vi "MEASURE_hysteresis_multiple_gate_Raman_all 2450.vi"() -> ()   [LabVIEW 2020]
uses:
  <vilib>/Utility/file.llb/Write To Spreadsheet File (DBL).vi
  C/Program Files/National Instruments/LabVIEW 2016/instr.lib/Stanford Research 830/Stanford Research 830.lvlib
  C/Program Files/National Instruments/LabVIEW 2016/instr.lib/Keithley 2450/Keithley 2450.lvlib
panel:
  out "back gate leaking":string="1.162721E-12\n"
  in  "Compliance  Level (1uA)":dbl=1e-09
  in  "Function (0: Volts) 3":u16(ring) items=["Volts", "Current", "Resistance"]
  in  "topgate-off set":dbl=3.0
  in  "0ff set{T}/no off set[F]":bool
  out "XY Graph 4":cluster{dbl[], dbl[]}(graph)
  out "XY Graph 3":cluster{dbl[], dbl[]}(graph)
  out "bottom gate voltage":dbl=0.22 format="%#_13g"
  in  "backgate address":refnum<visa-resource-name>="GPIB0::18::INSTR"
  in  "bottom gate thickness":dbl=30.0
  in  "top gate thickness":dbl=10.0
  in  "pure field (T)/pure doping (F)":bool=TRUE
  out "loop run":i32=1
  in  "loop #":i32=1
  in  "Save data or not":bool
  in  "path (folder + filename)":string="C:\\Users\\User\\Data\\Jason\\03282019\\ pure_bottom_high_6v_rato3 with light2"
  in  "Clear Plot":bool
  out "LOCKIN Measurement":dbl
  in  "Parameter (1: X)":u16(ring)=3 items=["X"=1, "Y"=2, "R"=3, "Theta"=4, "Channel 1"=5, "Channel 2"=6, "Aux In 1"=7, "Aux In 2"=8, "Aux In 3"=9, "Aux In 4"=10]
  out "top gate voltage":dbl=0.22 format="%#_13g"
  out "top gate leaking":string="-2.408176E-13\n"
  in  "GATE STEP(mv)":i32=50
  in  "GATE Low Value (default 0)":dbl
  in  "GATE High Value":dbl=0.5
  in  "Function (0: Volts) 2":u16(ring) items=["Volts", "Current", "Resistance"]
  in  "Source Compaliance":dbl=1e-09
  in  "topgate address":refnum<visa-resource-name>="GPIB0::18::INSTR"
  in  "SD stabilization(S) 2":dbl=0.3 format="%#_13g"
  in  "Sine Output Amplitude (1 V) 2":dbl=0.02
  in  "GATE / SD stablization 3":dbl=0.3 format="%#_13g"
  in  "frequency":dbl=50.0 format="%#_13g"
  in  "Input Connection (0: Single-Ended Voltage)":u16(ring)=1 items=["Single-Ended Voltage", "Differential Voltage", "1 MOhm Current Gain", "100 MOhm Current Gain"]
  in  "LOCKIN address":refnum<visa-resource-name>="GPIB0::8::INSTR"
  # "Gate2450 (back) Setting"
  # "Lock-in"
  # "Gate2450(top) Setting"
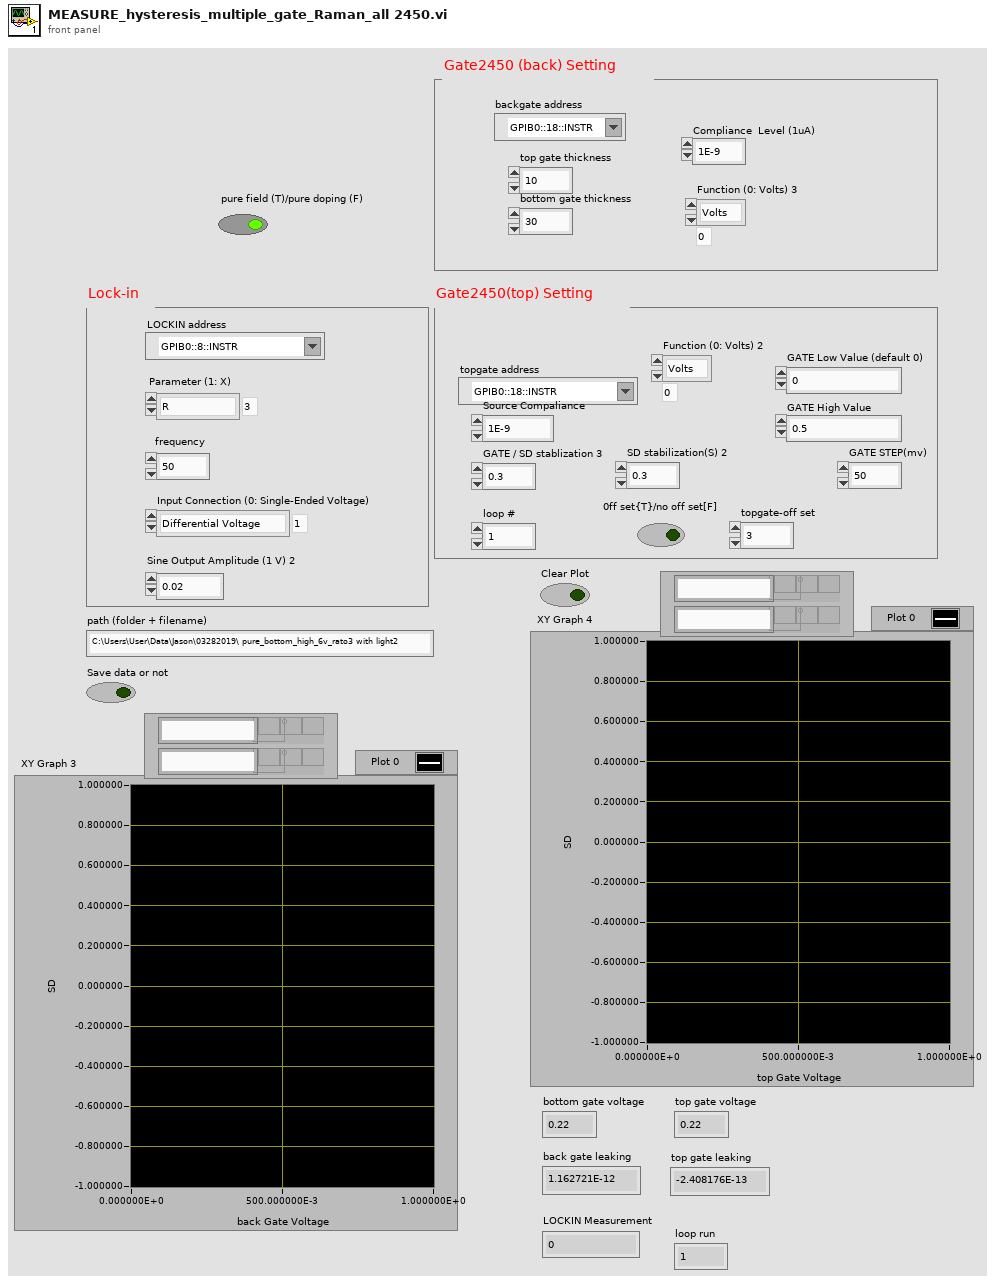
[diagram p1: front panel]
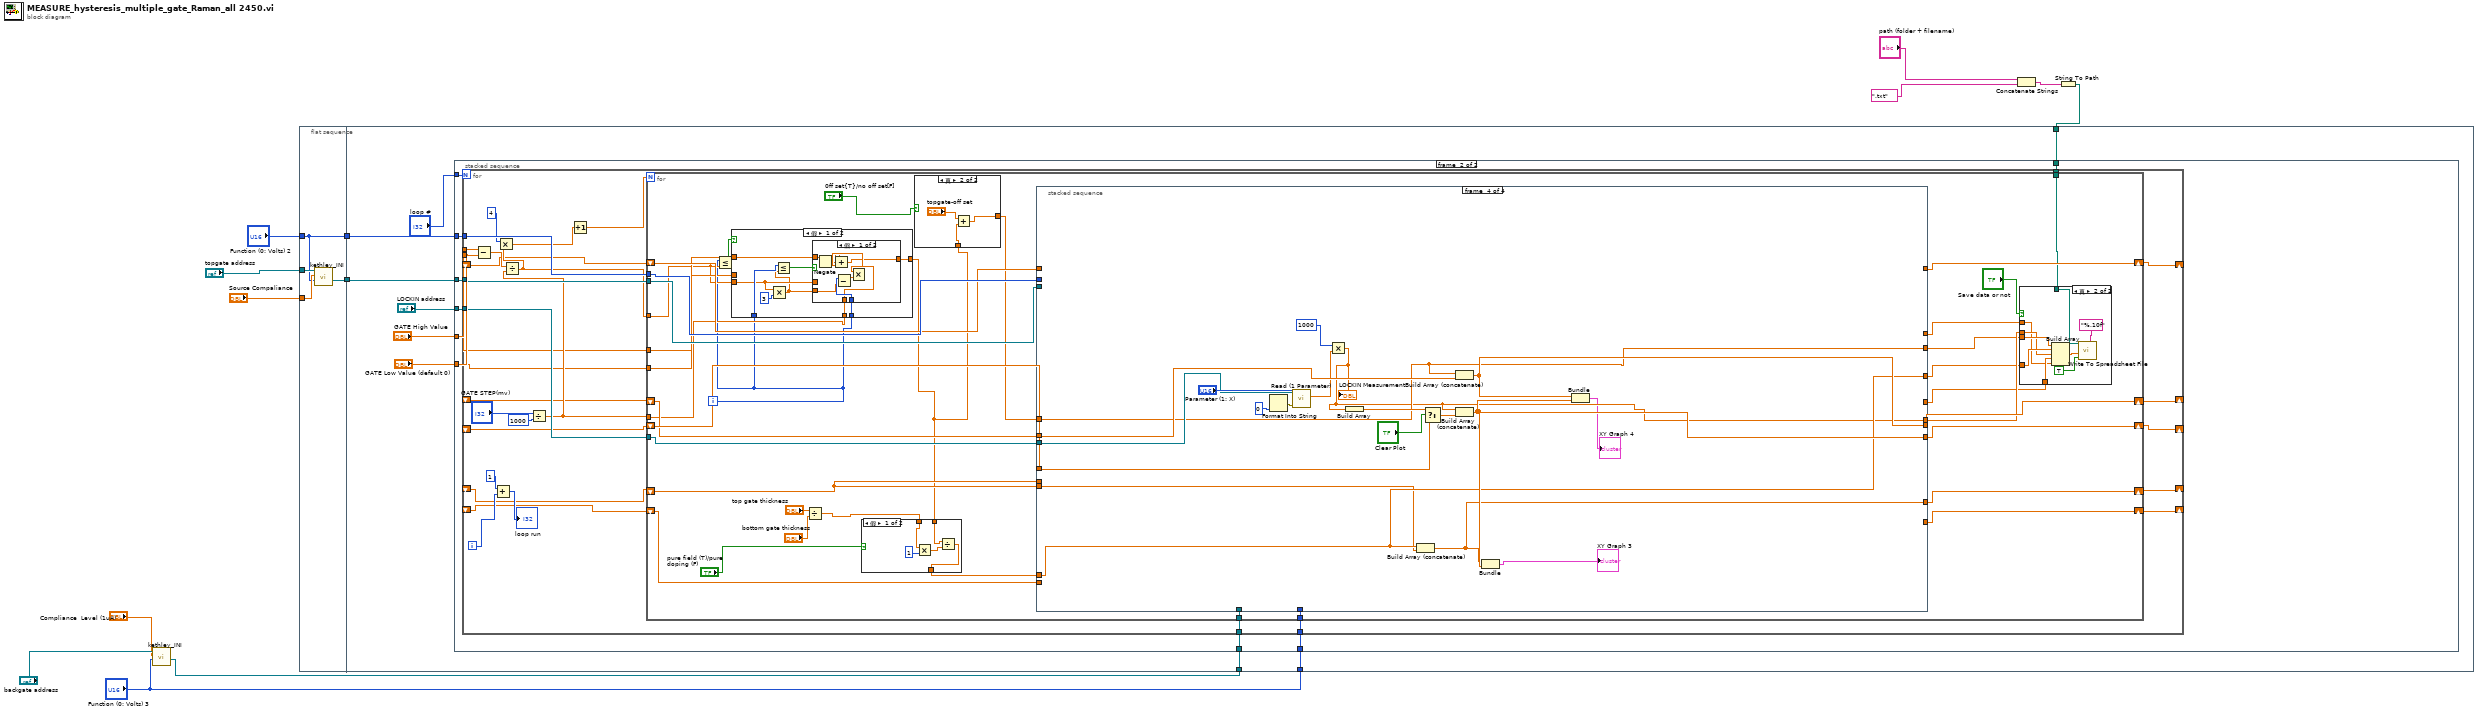
[diagram p0: block diagram]
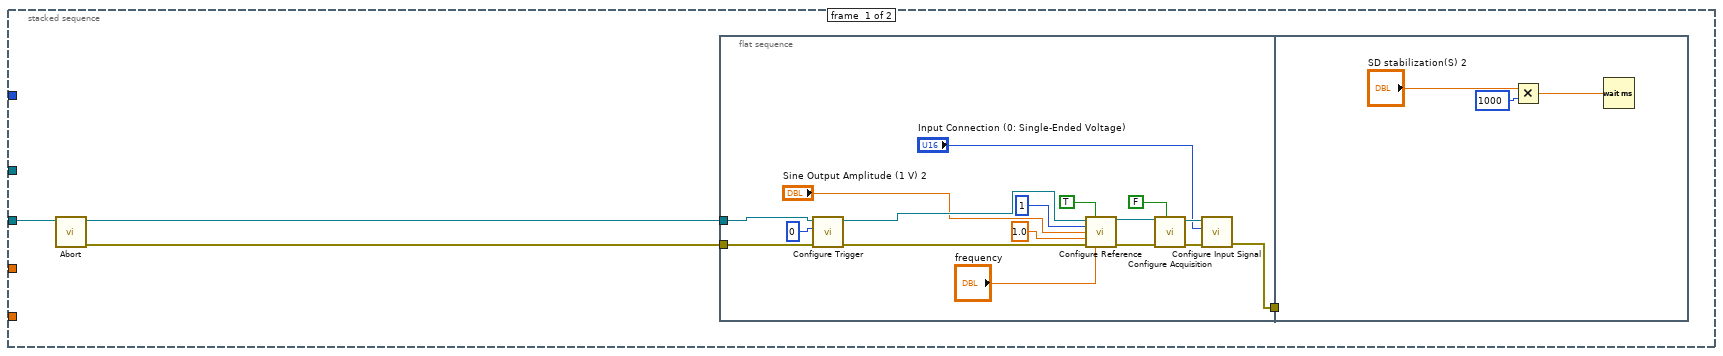
[diagram p2: hidden frame]
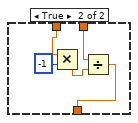
[diagram p4: hidden frame]
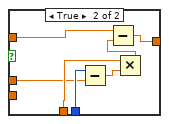
[diagram p6: hidden frame]
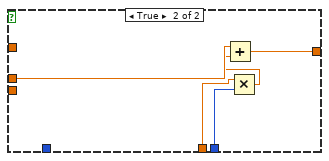
[diagram p7: hidden frame]
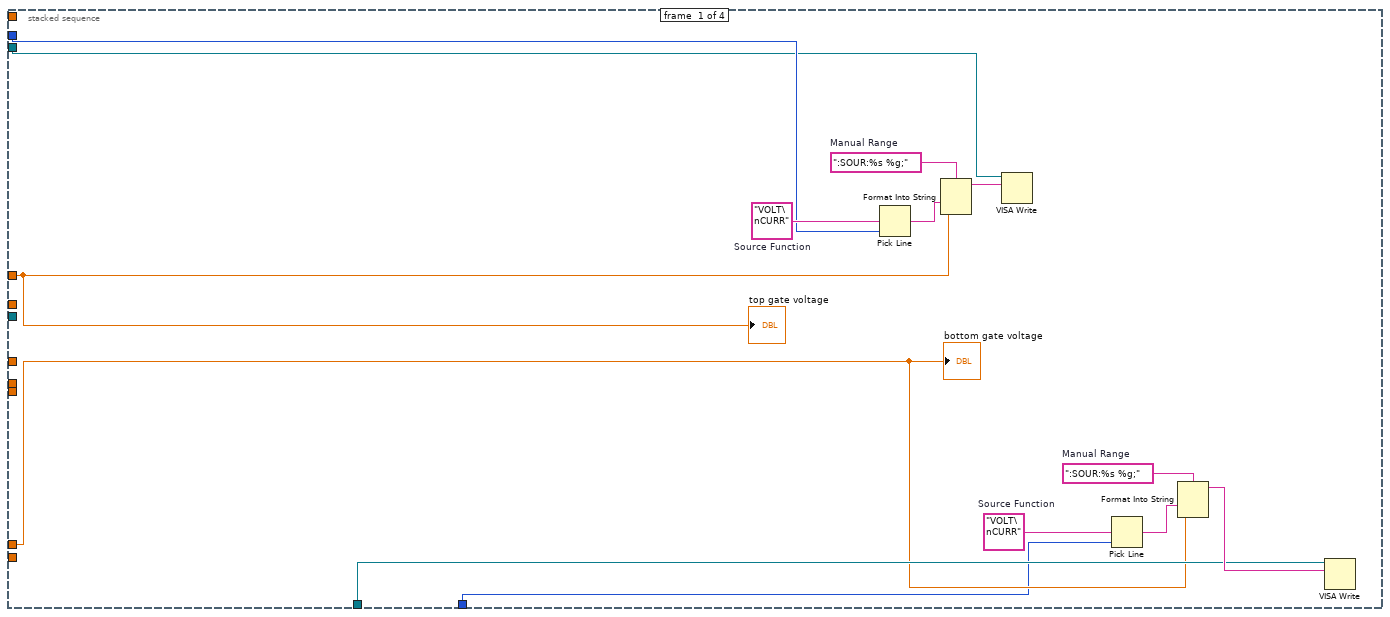
[diagram p8: hidden frame]
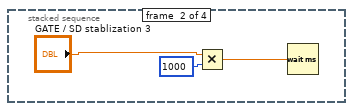
[diagram p9: hidden frame]
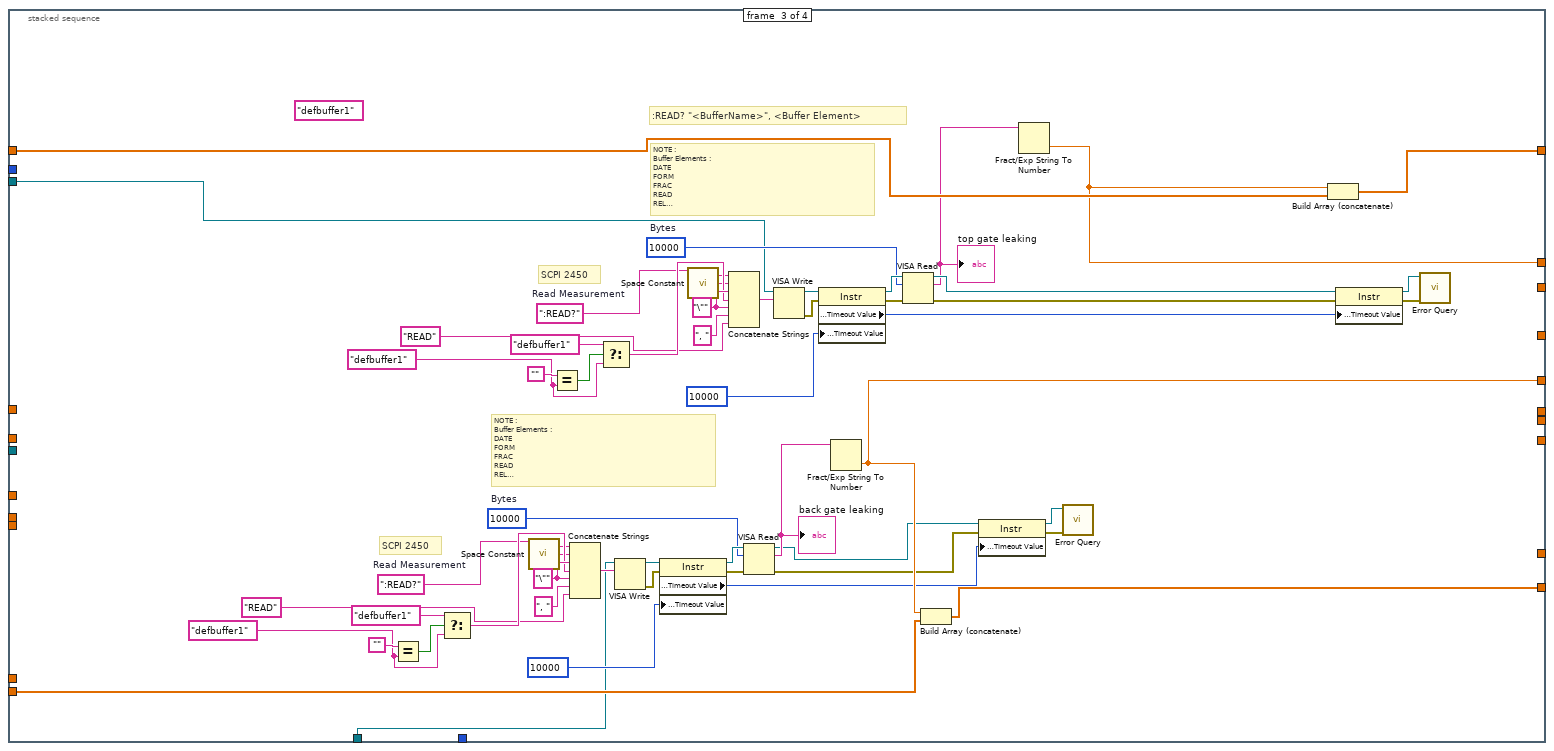
[diagram p10: hidden frame]
diagram:
  n1 = call "kethley_INI.vi"("Function (0: Volts) in"="Function (0: Volts) 3", "Source Compaliance"="Compliance  Level (1uA)", "VISA Refnum in"="backgate address") -> ("VISA resource name out"=w2:refnum<visa-resource-name>)  [unwired: 8 in]
  n2 = flat-sequence {
    tunnel: "topgate address" -> [w17]
    tunnel: "Source Compaliance" -> [w16]
    tunnel: "Function (0: Volts) 2" -> [w14]
    tunnel: [w15] -> w10
    tunnel: [w14] -> w9
    tunnel: w10 -> [w25]
    tunnel: w9 -> [w24]
    tunnel: w5 -> [w21]
    tunnel: w2 -> [w19]
    tunnel: "Function (0: Volts) 3" -> [w18]
    frame #0 {
      n3 = call "kethley_INI.vi"("Function (0: Volts) in"=w14, "Source Compaliance"=w16, "VISA Refnum in"=w17) -> ("VISA resource name out"=w15:refnum<visa-resource-name>)  [unwired: 8 in]
    }
    frame #1 {
      n4 = stacked-sequence {
        tunnel: "LOCKIN address" -> [w29 w57]
        tunnel: w25 -> [_ w58]
        tunnel: w24 -> [_ w59]
        tunnel: "GATE High Value" -> [_ w55]
        tunnel: "GATE Low Value (default 0)" -> [_ w56]
        tunnel: w21 -> [_ w54]
        tunnel: "loop #" -> [_ w53]
        tunnel: w19 -> [_ w52]
        tunnel: w18 -> [_ w51]
        frame #0 {
          n5 = call "Abort.vi"("VISA resource name"=w29) -> ("error out"=w27:errorcluster, "VISA resource name out"=w28:refnum<visa-resource-name>)  [unwired: 9 in]
          n6 = flat-sequence {
            tunnel: w28 -> [w47]
            tunnel: [w32] -> w30
            tunnel: w27 -> [w31]
            tunnel: w30 -> [_]
            frame #0 {
              n7 = call "Configure Trigger.vi"("error in (no error)"=w31, "Trigger Source (0: Internal)"=0, "VISA resource name"=w47) -> ("error out"=w41:errorcluster, "VISA resource name out"=w42:refnum<visa-resource-name>)  [unwired: 7 in]
              n8 = call "Configure Reference.vi"("VISA resource name"=w42, "Auto Phase (T: Enabled)"=TRUE, "Reference Source (1: Internal)"=1, "Sine Output Amplitude (1 V)"="Sine Output Amplitude (1 V) 2", "Detection Harmonic Number (1)"=1.0 ("output voltage 2"), "error in (no error)"=w41, "Internal Reference Frequency (1000 Hz)"="frequency") -> ("VISA resource name out"=w39:refnum<visa-resource-name>, "error out"=w34:errorcluster)  [unwired: 7 in]
              n9 = call "Configure Acquisition.vi"("Continuous Storage (T: Enable)"=FALSE, "error in (no error)"=w34, "VISA resource name"=w39) -> ("error out"=w33:errorcluster, "VISA resource name out"=w37:refnum<visa-resource-name>)  [unwired: 7 in]
              n10 = call "Configure Input Signal.vi"("error in (no error)"=w33, "Input Connection (0: Single-Ended Voltage)"="Input Connection (0: Single-Ended Voltage)", "VISA resource name"=w37) -> ("error out"=w32:errorcluster)  [unwired: 7 in, 1 out]
            }
            frame #1 {
              n11 = Multiply(x="SD stabilization(S) 2", y=1000) -> (x*y=w50:dbl)
              n12 = Wait (ms)(milliseconds to wait=w50) -> ()  [unwired: 1 out]
            }
          }
        }
        frame #1 {
          n13 = for {
            N: w53 -> [_]
            tunnel: w59 -> [w88]
            tunnel: w58 -> [w87]
            tunnel: w57 -> [w86]
            tunnel: w56 -> [w80]
            tunnel: w55 -> [w79]
            tunnel: w54 -> [w78]
            shift-right: [w74] -> _
            shift-left: _ -> [w73]
            shift-right: [w72] -> _
            shift-left: _ -> [w70]
            shift-right: [w71] -> _
            shift-left: _ -> [w69]
            shift-right: [w65] -> _
            shift-left: _ -> [w64]
            shift-right: [w63] -> _
            shift-left: _ -> [w62]
            tunnel: w52 -> [w61]
            tunnel: w51 -> [w60]
            i -> [w67]
            n14 = Subtract(x=w79, y=w80) -> (x-y=w82:dbl)
            n15 = Add(x=1, y=w67) -> (x+y=→"loop run":i32)
            n16 = Divide(x="GATE STEP(mv)", y=1000) -> (x/y=w81:dbl)
            n17 = Divide(x=w82, y=w81) -> (x/y=w77:dbl)
            n18 = Multiply(x=4, y=w77) -> (x*y=w76:dbl)
            n19 = Increment(x=w76) -> (x+1=w75:dbl)
            n20 = for {
              N: w75 -> [_]
              tunnel: w88 -> [w124]
              tunnel: w87 -> [w123]
              tunnel: w86 -> [w122]
              tunnel: w81 -> [w113]
              shift-right: [w121] -> w74
              shift-left: w73 -> [w120]
              shift-right: [w117] -> w71
              shift-left: w69 -> [w119]
              shift-right: [w116] -> w72
              shift-left: w70 -> [w118]
              tunnel: w77 -> [w111]
              tunnel: w80 -> [w114]
              tunnel: w79 -> [w112]
              tunnel: w78 -> [w106]
              shift-right: [w104] -> w65
              shift-left: w64 -> [w95]
              shift-right: [w103] -> w63
              shift-left: w62 -> [w94]
              tunnel: w61 -> [w101]
              tunnel: w60 -> [w89]
              i -> [w110]
              n21 = Less Or Equal?(x=w110, y=w111) -> (x <= y?=w115:bool)
              n22 = case shown="假" w115 {
                tunnel: w114 -> [_ w176]
                tunnel: w110 -> [w156 w175]
                tunnel: w113 -> [w155 w174]
                tunnel: [w153 w172] -> w91
                tunnel: w112 -> [w154 _]
                tunnel: w111 -> [w149 _]
                tunnel: w110 -> [w152 _]
                frame False {
                  n23 = Multiply(x=w149, y=3) -> (x*y=w148:dbl)
                  n24 = Less Or Equal?(x=w152, y=w148) -> (x <= y?=w150:bool)
                  n25 = case shown="假" w150 {
                    tunnel: w156 -> [w164 w171]
                    tunnel: w155 -> [w162 w169]
                    tunnel: w154 -> [w158 w167]
                    tunnel: [w160 w166] -> w153
                    tunnel: w149 -> [_ w165]
                    tunnel: w148 -> [w157 _]
                    frame False {
                      n26 = Negate(x=w158) -> (-x=w159:dbl)
                      n27 = Subtract(x=w164, y=w157) -> (x-y=w163:dbl)
                      n28 = Multiply(x=w162, y=w163) -> (x*y=w161:dbl)
                      n29 = Add(x=w159, y=w161) -> (x+y=w160:dbl)
                    }
                    frame True {
                      n30 = Subtract(x=w171, y=w165) -> (x-y=w170:dbl)
                      n31 = Multiply(x=w169, y=w170) -> (x*y=w168:dbl)
                      n32 = Subtract(x=w167, y=w168) -> (x-y=w166:dbl)
                    }
                  }
                }
                frame True {
                  n33 = Multiply(x=w174, y=w175) -> (x*y=w173:dbl)
                  n34 = Add(x=w176, y=w173) -> (x+y=w172:dbl)
                }
              }
              n35 = Divide(x="top gate thickness", y="bottom gate thickness") -> (x/y=w100:dbl)
              n36 = case shown="假" "pure field (T)/pure doping (F)" {
                tunnel: w100 -> [w132 w138]
                tunnel: [w129 w136] -> w96
                tunnel: w91 -> [w130 w135]
                frame False {
                  n37 = Multiply(x=w132, y=1) -> (x*y=w131:dbl)
                  n38 = Divide(x=w130, y=w131) -> (x/y=w129:dbl)
                }
                frame True {
                  n39 = Multiply(x=w138, y=-1) -> (x*y=w134:dbl)
                  n40 = Divide(x=w135, y=w134) -> (x/y=w136:dbl)
                }
              }
              n41 = case shown="真" "0ff set{T}/no off set[F]" {
                tunnel: w91 -> [w125 w128]
                tunnel: [w125 w126] -> w90
                frame False {
                }
                frame True {
                  n42 = Add(x="topgate-off set", y=w128) -> (x+y=w126:dbl)
                }
              }
              n43 = stacked-sequence {
                tunnel: w124 -> [w186 _ _ _]
                tunnel: w123 -> [w185 _ w225 _]
                tunnel: w122 -> [_ _ _ w259]
                tunnel: w90 -> [w184 _ _ w258]
                tunnel: [_ _ w223 _] -> w121
                tunnel: w120 -> [_ _ w224 _]
                tunnel: w119 -> [_ _ _ w262]
                tunnel: w118 -> [_ _ _ w260]
                tunnel: [_ _ _ w255] -> w117
                tunnel: [_ _ _ w261] -> w116
                tunnel: [_ _ _ w249] -> w109
                tunnel: [_ _ _ w258] -> w108
                tunnel: [_ _ w221 _] -> w107
                tunnel: [_ _ w220 _] -> w104
                tunnel: [_ _ _ w254] -> w103
                tunnel: w94 -> [_ _ _ _]
                tunnel: [_ _ _ w253] -> w102
                tunnel: [_ _ w199 _] -> w93
                tunnel: w101 -> [w179 _ w201 _]
                tunnel: w96 -> [w178 _ _ w253]
                tunnel: w95 -> [_ _ w219 _]
                tunnel: w94 -> [_ _ _ w252]
                tunnel: w89 -> [w177 _ _ _]
                frame #0 {
                  w181 = "VOLT\nCURR"  # Source Function
                  w182 = ":SOUR:%s %g;"  # Manual Range
                  w188 = "VOLT\nCURR"  # Source Function
                  w189 = ":SOUR:%s %g;"  # Manual Range
                  n44 = Pick Line(multi-line string=w188, line index=w186) -> (output string=w187:string)  [unwired: 1 out]
                  n45 = Format Into String(format string=w189, w187, w184) -> (resulting string=w190:string)  [unwired: 2 in, 1 out]
                  n46 = VISA Write(VISA resource name=w185, write buffer=w190) -> ()  [unwired: 1 in, 3 out]
                  n47 = Pick Line(multi-line string=w181, line index=w177) -> (output string=w180:string)  [unwired: 1 out]
                  n48 = Format Into String(format string=w182, w180, w178) -> (resulting string=w183:string)  [unwired: 2 in, 1 out]
                  n49 = VISA Write(VISA resource name=w179, write buffer=w183) -> ()  [unwired: 1 in, 3 out]
                  "top gate voltage" <- w184
                  "bottom gate voltage" <- w178
                }
                frame #1 {
                  n50 = Multiply(x="GATE / SD stablization 3", y=1000) -> (x*y=w193:dbl)
                  n51 = Wait (ms)(milliseconds to wait=w193) -> ()  [unwired: 1 out]
                }
                frame #2 {
                  w210 = "defbuffer1" ("Buffer Name (defbuffer1) 2")
                  w208 = "\""
                  w205 = ":READ?"  # Read Measurement
                  w214 = u32 10000  # Bytes
                  w236 = "defbuffer1" ("Buffer Name (defbuffer1) 2")
                  (unwired) "defbuffer1" ("t")
                  w234 = "\""
                  w231 = ":READ?"  # Read Measurement
                  w240 = u32 10000  # Bytes
                  # "NOTE :\nBuffer Elements :\nDATE\nFORM\nFRAC\nREAD\nREL\nSEC\nSOUR\nSOURFORM\nSOURSTAT\nSOURUNIT\nSTAT\nTIME\nTsT\nUNIT"
                  # "SCPI 2450"
                  # "NOTE :\nBuffer Elements :\nDATE\nFORM\nFRAC\nREAD\nREL\nSEC\nSOUR\nSOURFORM\nSOURSTAT\nSOURUNIT\nSTAT\nTIME\nTsT\nUNIT"
                  # ":READ? \"<BufferName>\", <Buffer Element>"
                  # "SCPI 2450"
                  n52 = Equal?(x="", y=w210) -> (x = y?=w211:bool)
                  n53 = Select(t="defbuffer1", s=w211, f=w210) -> (s? t:f=w207:string)
                  n54 = call <vilib>:"Space Constant.vi"() -> ("String"=w206:string)
                  n55 = Equal?(x="", y=w236) -> (x = y?=w237:bool)
                  n56 = Concatenate Strings(w205, w206, w208, w207, w208, ", " ("string"), "READ" ("Buffer Elements 2")) -> (w218:string)
                  n57 = Select(t="defbuffer1", s=w237, f=w236) -> (s? t:f=w233:string)
                  n58 = VISA Write(VISA resource name=w201, write buffer=w218) -> (VISA resource name out=w213:refnum<visa-resource-name>, error out=w217:errorcluster)  [unwired: 1 in, 1 out]
                  n59 = property class="Instr"(reference=w213, error in=w217, "General Settings:Timeout Value"=10000 ("Timeout (10000 ms) 2")) -> (reference out=w216:refnum<visa-resource-name>, error out=w215:errorcluster, "General Settings:Timeout Value"=w194:u32)
                  n60 = call <vilib>:"Space Constant.vi"() -> ("String"=w232:string)
                  n61 = Concatenate Strings(w231, w232, w234, w233, w234, ", " ("string"), "READ" ("Buffer Elements 2")) -> (w247:string)
                  n62 = VISA Read(VISA resource name=w216, byte count=w214, error in (no error)=w215) -> (VISA resource name out=w195:refnum<visa-resource-name>, read buffer=w200:string, error out=w196:errorcluster)  [unwired: 1 out]
                  "back gate leaking" <- w200
                  n63 = VISA Write(VISA resource name=w225, write buffer=w247) -> (VISA resource name out=w239:refnum<visa-resource-name>, error out=w246:errorcluster)  [unwired: 1 in, 1 out]
                  n64 = property class="Instr"(reference=w239, error in=w246, "General Settings:Timeout Value"=10000 ("Timeout (10000 ms) 2")) -> (reference out=w245:refnum<visa-resource-name>, error out=w244:errorcluster, "General Settings:Timeout Value"=w241:u32)
                  n65 = Fract/Exp String To Number(string=w200) -> (number=w199:dbl)  [unwired: 3 in, 1 out]
                  n66 = VISA Read(VISA resource name=w245, byte count=w240, error in (no error)=w244) -> (VISA resource name out=w243:refnum<visa-resource-name>, read buffer=w222:string, error out=w242:errorcluster)  [unwired: 1 out]
                  "top gate leaking" <- w222
                  n67 = Build Array (concatenate)(w199, w219) -> (w220:dbl[])
                  n68 = property class="Instr"(reference=w195, error in=w196, "General Settings:Timeout Value"=w194) -> (reference out=w198:refnum<visa-resource-name>, error out=w197:errorcluster)
                  n69 = Fract/Exp String To Number(string=w222) -> (number=w221:dbl)  [unwired: 3 in, 1 out]
                  n70 = call "Error Query.vi"("error in (no error)"=w197, "VISA resource name"=w198) -> ()  [unwired: 10 out]
                  n71 = Build Array (concatenate)(w221, w224) -> (w223:dbl[])
                  n72 = property class="Instr"(reference=w243, error in=w242, "General Settings:Timeout Value"=w241) -> (reference out=w229:refnum<visa-resource-name>, error out=w228:errorcluster)
                  n73 = call "Error Query.vi"("error in (no error)"=w228, "VISA resource name"=w229) -> ()  [unwired: 10 out]
                }
                frame #3 {
                  n74 = Format Into String(0) -> (error out=w267:errorcluster)  [unwired: 3 in, 1 out]
                  n75 = call "Read (1 Parameter).vi"("error in (no error)"=w267, "Parameter (1: X)"="Parameter (1: X)", "VISA resource name"=w259) -> ("Measurement"=w250:dbl)  [unwired: 6 in, 2 out]
                  n76 = Multiply(x=1000, y=w250) -> (x*y=w249:dbl)
                  "LOCKIN Measurement" <- w249
                  n77 = Build Array(w249) -> (w265:dbl[])
                  n78 = Build Array (concatenate)(w253, w252) -> (w254:dbl[])
                  n79 = Select(t=w265, s="Clear Plot", f=w262) -> (s? t:f=w257:dbl[])
                  n80 = Build Array (concatenate)(w258, w260) -> (w261:dbl[])
                  n81 = Build Array (concatenate)(w249, w257) -> (w255:dbl[])
                  n82 = Bundle(w254, w255) -> (→"XY Graph 3":cluster{dbl[], dbl[]})  [unwired: 1 in]
                  n83 = Bundle(w261, w255) -> (→"XY Graph 4":cluster{dbl[], dbl[]})  [unwired: 1 in]
                }
              }
              n84 = case shown="真" "Save data or not" {
                tunnel: w109 -> [_ w140]
                tunnel: w108 -> [_ w147]
                tunnel: w107 -> [_ w139]
                tunnel: w106 -> [_ w145]
                tunnel: w102 -> [_ w141]
                tunnel: w93 -> [_ w142]
                frame False {
                }
                frame True {
                  n85 = Build Array(w147, w141, w140, w142, w139) -> (w146:dbl[])
                  n86 = call-poly <vilib>:"Write To Spreadsheet File.vi"("format (%.3f)"="%.10f", "append to file? (new file:F)"=TRUE, "1D data"=w146, "file path (dialog if empty)"=w145) -> ()  [unwired: 4 in, 1 out]
                }
              }
            }
          }
        }
      }
    }
  }
  n87 = Concatenate Strings("path (folder + filename)", ".txt") -> (w6:string)
  n88 = String To Path(string=w6) -> (path=w5:path)
